vi "Get Hardware Relay State.vi"(0 "RelayInterface in":refnum<class "RelayInterface.lvclass">, 5 "session in":refnum<k21>, 7 "device in":refnum<k21>, 11 "error in (no error)":errorcluster) -> (4 "RelayInterface out":refnum<class "RelayInterface.lvclass">, 6 "session out":refnum<k21>, 8 "device out":refnum<k21>, 10 "RelayPosition":T1=10 caption="position" items=["Open"=10, "Closed"=11], 15 "error out":errorcluster)   [LabVIEW 2015, in "RelayInterface.lvclass"]
uses:
  RelayInterface.lvclass
  slscsl/RelayPosition.ctl
  slscsl/slscsl.lvclass
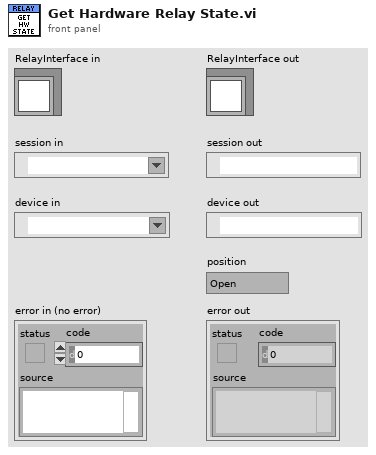
[diagram p1: front panel]
types:
  T1 = typedef "slscsl.lvclass/RelayPosition.ctl" = i32
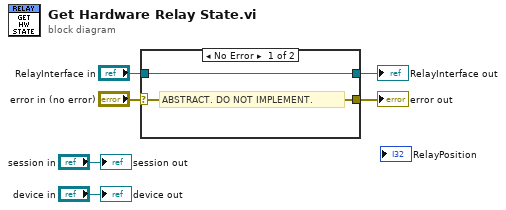
[diagram p0: block diagram]
diagram:
  n1 = case shown="No Error" "error in (no error)" {
    selector: "error in (no error)" -> [w8 w10]
    tunnel: [w8 w10] -> w5
    tunnel: [w7 w9] -> w3
    tunnel: "RelayInterface in" -> [w7 w9]
    frame No Error {
      # "ABSTRACT. DO NOT IMPLEMENT."
    }
    frame Error {
    }
  }
  "error out" <- w5
  "RelayInterface out" <- w3
  "device out" <- "device in"
  "session out" <- "session in"
